vi "Add Cell.vi"(6 "Reinsert?":bool, 8 "error in (no error)":errorcluster, 10 "Schedule Cell":refnum<class "Schedule Cell.lvclass">, 11 "Schedule in":refnum<class "Schedule.lvclass">) -> (0 "error out":errorcluster, 3 "Schedule out":refnum<class "Schedule.lvclass">)   [LabVIEW 2020, in "TALOS.lvlib" / "Run Utilities.lvlib" / "Schedule.lvclass"]
doc: "Vi for adding new Run Instance into the schedule. It appends the value to the existing array"
uses:
  Schedule.lvclass
  Cell/Schedule Cell.lvclass
  Run Instance/Run Instance.lvclass
  Schedule.lvclass/Schedule.ctl
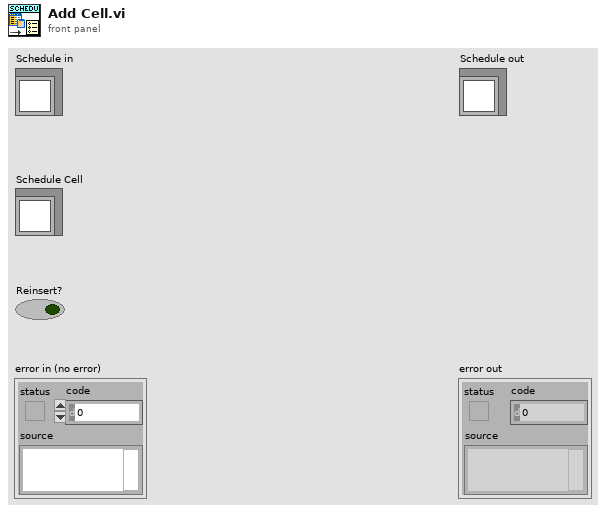
[diagram p1: front panel]
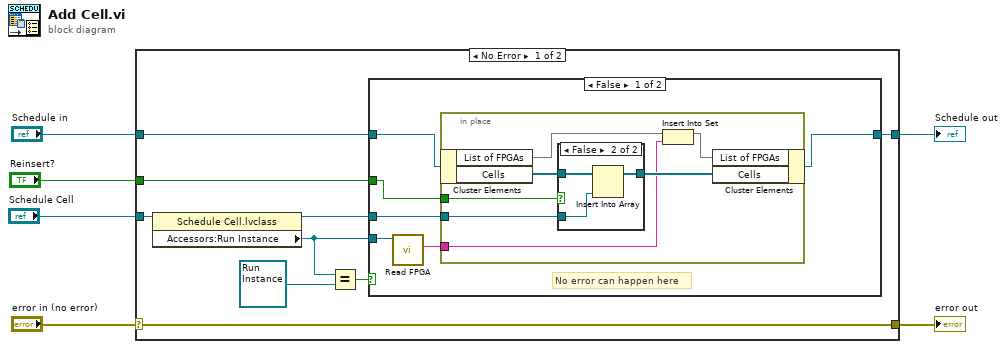
[diagram p0: block diagram]
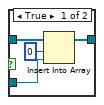
[diagram p2: hidden frame]
diagram:
  n1 = case shown="No Error" "error in (no error)" {
    selector: "error in (no error)" -> [w10 w38]
    tunnel: [w10 w38] -> w5
    tunnel: [w14 w37] -> w3
    tunnel: "Schedule in" -> [w15 w37]
    tunnel: "Schedule Cell" -> [w11 _]
    tunnel: "Reinsert?" -> [w7 _]
    frame No Error {
      n2 = property class="Schedule Cell.lvclass"(reference=w11) -> (reference out=w9:refnum<class "Schedule Cell.lvclass">, "Accessors:Run Instance"=w8:refnum<class "Run Instance.lvclass">)  [unwired: 1 in, 1 out]
      n3 = Equal?(x=w8, y=refnum<class "Run Instance.lvclass"> refnum ("Run Instance")) -> (x = y?=w12:bool)
      n4 = case shown="False" w12 {
        tunnel: w15 -> [w18 w36]
        tunnel: [w16 w36] -> w14
        tunnel: w8 -> [w21 _]
        tunnel: w9 -> [w19 _]
        tunnel: w7 -> [w20 _]
        frame False {
          # "No error can happen here"
          n5 = call-dynamic "Read FPGA.vi"("Run Instance in"=w21) -> ("FPGA Name"=w17:string)  [unwired: 8 in, 2 out]
          n6 = in-place {
            in-place-border: w20 -> [w28]
            in-place-border: w19 -> [w27]
            in-place-border: w17 -> [w24]
            n7 = in-place-cluster #1(w18) -> ("List of FPGAs"=w23:set{string}, "Cells"=w26:refnum<class "Schedule Cell.lvclass">[])
            n8 = case shown="False" w28 {
              tunnel: w26 -> [w32 w35]
              tunnel: [w31 w34] -> w25
              tunnel: w27 -> [w29 w33]
              frame True {
                n9 = Insert Into Array(array=w32, index=0, new element=w29) -> (w31:refnum<class "Schedule Cell.lvclass">[])
              }
              frame False {
                n10 = Insert Into Array(array=w35, new element=w33) -> (w34:refnum<class "Schedule Cell.lvclass">[])  [unwired: 1 in]
              }
            }
            n11 = Insert Into Set(10:w24, 11:w23) -> (3:w22:set{string})  [unwired: 1 out]
            n12 = in-place-cluster #1("List of FPGAs"=w22, "Cells"=w25) -> (w16:refnum<class "Schedule.lvclass">)
          }
        }
        frame True {
          # "Run Instance is empty, do nothing"
        }
      }
    }
    frame Error {
    }
  }
  "error out" <- w5
  "Schedule out" <- w3
